vi "Read U8 From 1 Address.vi"(8 "error in (no error)":errorcluster, 9 "Address number (0)":u8 max=49, 10 "Motor ID (0)":u8, 11 "Dynamixel Motor VISA in":refnum<class "Dynamixel Motor VISA.lvclass">) -> (0 "error out":errorcluster, 2 "Data":u8, 3 "Dynamixel Motor VISA out":refnum<class "Dynamixel Motor VISA.lvclass">)   [LabVIEW 2016, in "Dynamixel Motor VISA.lvclass"]
doc: "Reads a single value/address from the motor's register. This is a Low-Level VI that is used by other VIs."
uses:
  <instrlib>/Dynamixel Motor/HAIOL/VISA/Dynamixel Motor VISA.lvclass
  <instrlib>/Dynamixel Motor/HAIOL/VISA/Dynamixel Motor VISA.lvclass/Dynamixel Motor VISA.ctl
  <instrlib>/Dynamixel Motor/Dynamixel Motor.lvlib
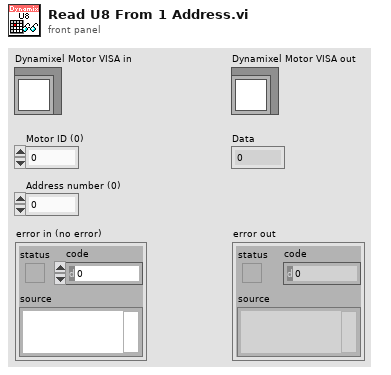
[diagram p1: front panel]
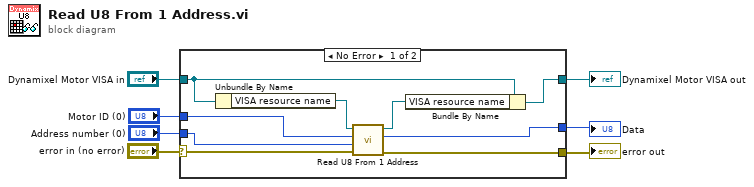
[diagram p0: block diagram]
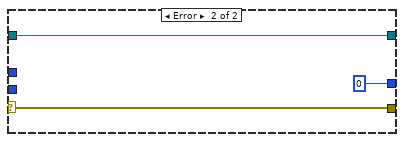
[diagram p2: hidden frame]
diagram:
  n1 = case shown="No Error" "error in (no error)" {
    selector: "error in (no error)" -> [w16 w18]
    tunnel: "Dynamixel Motor VISA in" -> [w10 w19]
    tunnel: "Motor ID (0)" -> [w14 _]
    tunnel: "Address number (0)" -> [w13 _]
    tunnel: [w12 w18] -> w3
    tunnel: [w9 w19] -> w2
    tunnel: [w8 u8 0 ("Data")] -> w1
    frame No Error {
      n2 = Unbundle By Name(w10) -> ("VISA resource name"=w15:refnum<visa-resource-name>)
      n3 = call <instrlib>:"Read U8 From 1 Address.vi"("Error in (no error)"=w16, "Address number (0)"=w13, "Motor ID (0)"=w14, "VISA resource name"=w15) -> ("error out"=w12:errorcluster, "Data"=w8:u8, "VISA resource name out"=w11:refnum<visa-resource-name>)  [unwired: 5 in]
      n4 = Bundle By Name(cluster=w10, "VISA resource name"=w11) -> (w9:refnum<class "Dynamixel Motor VISA.lvclass">)
    }
    frame Error {
    }
  }
  "error out" <- w3
  "Dynamixel Motor VISA out" <- w2
  "Data" <- w1
